vi "Status.vi"(8 "error in (no error)":errorcluster, 11 "Timer in":refnum<class "Timer.lvclass">) -> (0 "error out":errorcluster, 1 "Start?":bool, 2 "TimePeroid(ms)":i64, 3 "Timer out":refnum<class "Timer.lvclass">, 4 "EclipsedTime(ms)":i64)   [LabVIEW 2017, in "TimerEngine.lvlib" / "Timer.lvclass"]
uses:
  Timer.lvclass
  Timer.lvclass/Timer.ctl
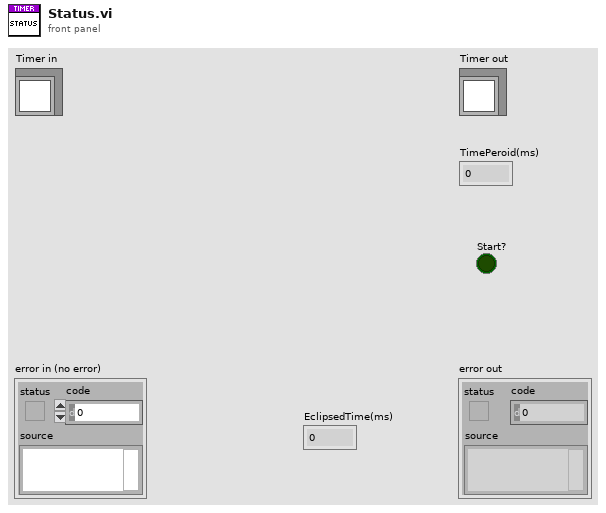
[diagram p1: front panel]
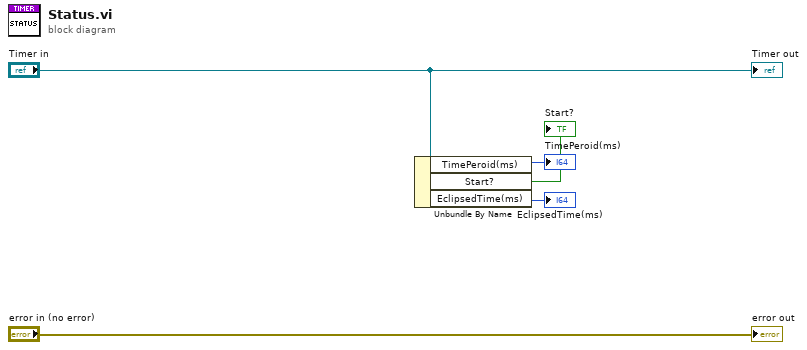
[diagram p0: block diagram]
diagram:
  n1 = Unbundle By Name("Timer in") -> ("TimePeroid(ms)"=→"TimePeroid(ms)":i64, "Start?"=→"Start?":bool, "EclipsedTime(ms)"=→"EclipsedTime(ms)":i64)
  "error out" <- "error in (no error)"
  "Timer out" <- "Timer in"
